vi "Determine if the Windows Environment is 32-bit or 64-bit 2017.vi"(8 "error in":errorcluster) -> (0 "error out":errorcluster, 1 "64-bit system":bool)   [LabVIEW 2018]
panel:
  out "32-bit system":bool
  out "CMD Output":string="This is the output from Windows Command Prompt. "
  out "String before \"-bit\"":string="This the same output, but only the portion before \"-bit\" in the original output. "
  out "32/64 subset":string="Substring containing \"32\" or \"64\""
  # "Overview: This VI uses parses the string output of the System Exec VI to determine if the Windows Environment is 32-bit or 64-bit.\nRequirement: LabVIEW 2012 or compatible\nInstructions:\n1. Run the VI.\n2. Check the lights to see if it is 32/64 bit OS"
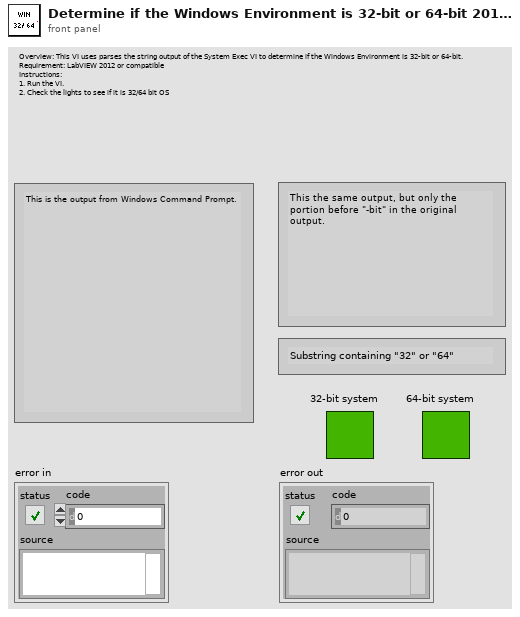
[diagram p1: front panel]
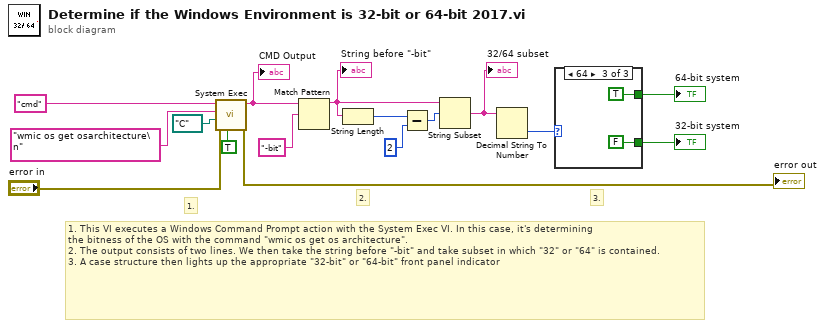
[diagram p0: block diagram]
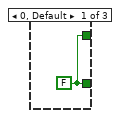
[diagram p2: hidden frame]
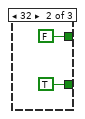
[diagram p3: hidden frame]
diagram:
  # "1. This VI executes a Windows Command Prompt action with the System Exec VI. In this case, it's determining \nthe bitness of the OS with the command \"wmic os get os architecture\".  \n2. The output consists of two lines. We then take the string before \"-bit\" and take subset in which \"32\" or \"64\" is contained.  \n3. A case structure then lights up the appropriate \"32-bit\" or \"64-bit\" front panel indicator"
  # "3."
  # "2."
  # "1."
  n1 = call <vilib>:"System Exec.vi"("run minimized? (F)"=TRUE, "error in (no error)"="error in", "working directory"=path "C:/", "standard input"="wmic os get osarchitecture\n", "command line"="cmd") -> ("error out"=→"error out":errorcluster, "standard output"=w5:string)  [unwired: 3 in, 2 out]
  "CMD Output" <- w5
  n2 = Match Pattern(string=w5, regular expression="-bit") -> (before substring=w6:string)  [unwired: 1 in, 3 out]
  "String before \"-bit\"" <- w6
  n3 = String Length(string=w6) -> (length=w11:i32)
  n4 = Subtract(x=w11, y=2) -> (x-y=w9:i32)
  n5 = String Subset(string=w6, offset (0)=w9) -> (substring=w7:string)  [unwired: 1 in]
  "32/64 subset" <- w7
  n6 = Decimal String To Number(string=w7) -> (number=w8:i32)  [unwired: 2 in, 1 out]
  n7 = case shown="64" w8 {
    tunnel: [w17 FALSE TRUE] -> w4
    tunnel: [w17 TRUE FALSE] -> w3
    frame 0, Default {
      w17 = FALSE
    }
    frame 32 {
    }
    frame 64 {
    }
  }
  "32-bit system" <- w3
  "64-bit system" <- w4
